vi "YZ_Stage_Movement.vi"(9 "Z Input":dbl, 10 "Y Input":dbl, 11 "X Input":dbl) -> (1 "Current Z Position":sgl, 2 "Current Y Position":sgl, 3 "Current X Position":sgl)   [LabVIEW 2013]
panel:
  out "Original Z Position":sgl
  out "Original Y Position":sgl
  out "Original X Position":sgl
  in  "Z Stage Serial":i32
  in  "Y Stage Serial":i32
  in  "X Stage Serial":i32
  in  "Z Stage Motor":refnum<k7>(container)
  in  "Y Stage Motor":refnum<k7>(container)
  in  "X Stage motor":refnum<k7>(container)
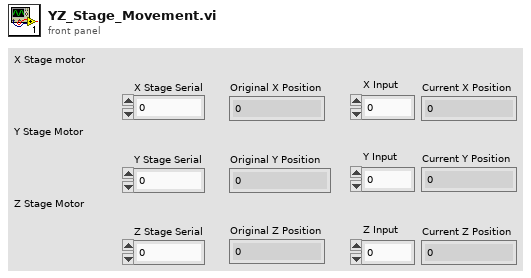
[diagram p1: front panel]
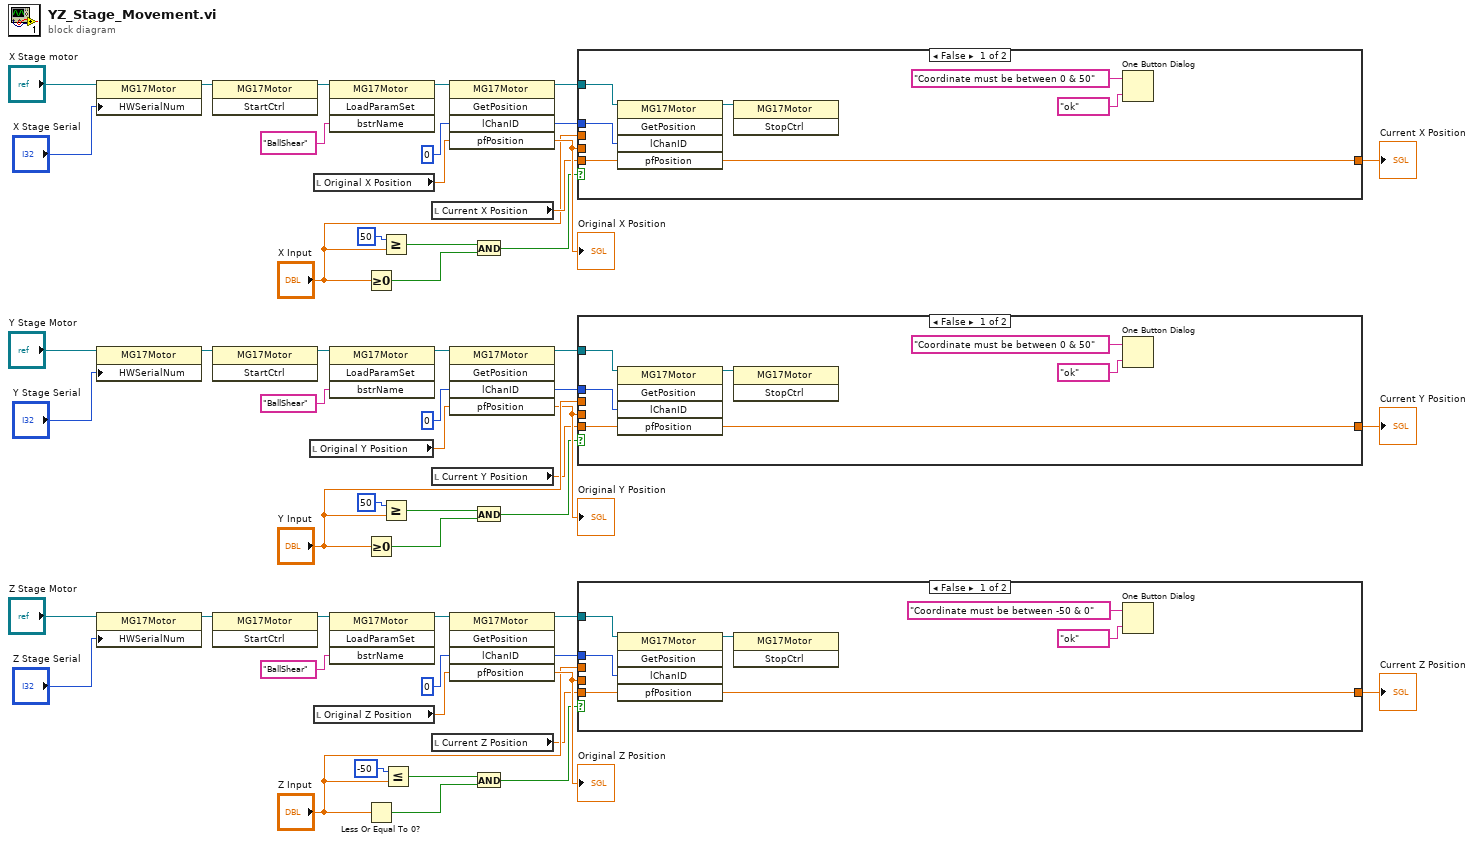
[diagram p0: block diagram]
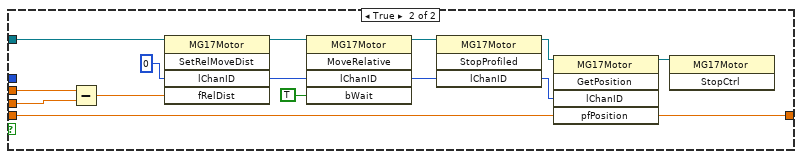
[diagram p2: hidden frame]
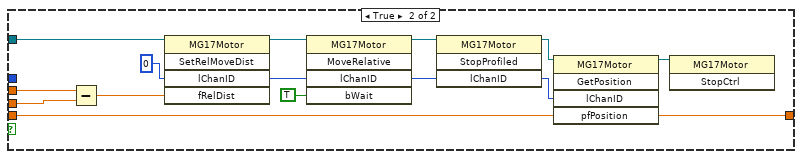
[diagram p3: hidden frame]
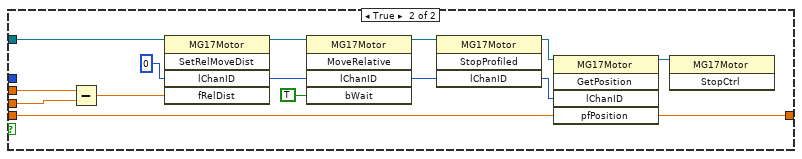
[diagram p4: hidden frame]
diagram:
  n1 = property class="MG17Motor"(reference="X Stage motor", "HWSerialNum"="X Stage Serial") -> (reference out=w46:refnum<k7>)  [unwired: 1 in, 1 out]
  n2 = property class="MG17Motor"(reference="Y Stage Motor", "HWSerialNum"="Y Stage Serial") -> (reference out=w47:refnum<k7>)  [unwired: 1 in, 1 out]
  n3 = property class="MG17Motor"(reference="Z Stage Motor", "HWSerialNum"="Z Stage Serial") -> (reference out=w48:refnum<k7>)  [unwired: 1 in, 1 out]
  n4 = invoke class="MG17Motor" method="StartCtrl"(reference=w46) -> (reference out=w16:refnum<k7>)  [unwired: 2 in, 2 out]
  n5 = invoke class="MG17Motor" method="StartCtrl"(reference=w47) -> (reference out=w13:refnum<k7>)  [unwired: 2 in, 2 out]
  n6 = invoke class="MG17Motor" method="StartCtrl"(reference=w48) -> (reference out=w18:refnum<k7>)  [unwired: 2 in, 2 out]
  n7 = local read "Original Y Position"() -> (w36:sgl)
  n8 = local read "Original X Position"() -> (w44:sgl)
  n9 = local read "Original Z Position"() -> (w28:sgl)
  n10 = invoke class="MG17Motor" method="LoadParamSet"(reference=w16, "bstrName"="BallShear") -> (reference out=w15:refnum<k7>)  [unwired: 2 in, 3 out]
  n11 = invoke class="MG17Motor" method="LoadParamSet"(reference=w13, "bstrName"="BallShear") -> (reference out=w12:refnum<k7>)  [unwired: 2 in, 3 out]
  n12 = invoke class="MG17Motor" method="LoadParamSet"(reference=w18, "bstrName"="BallShear") -> (reference out=w19:refnum<k7>)  [unwired: 2 in, 3 out]
  n13 = Greater Or Equal To 0?(x="X Input") -> (x >= 0?=w43:bool)
  n14 = Greater Or Equal To 0?(x="Y Input") -> (x >= 0?=w35:bool)
  n15 = Less Or Equal To 0?(x="Z Input") -> (x <= 0?=w21:bool)
  n16 = Greater Or Equal?(x=50, y="X Input") -> (x >= y?=w42:bool)
  n17 = Greater Or Equal?(x=50, y="Y Input") -> (x >= y?=w34:bool)
  n18 = Less Or Equal?(x=-50, y="Z Input") -> (x <= y?=w23:bool)
  n19 = local read "Current X Position"() -> (w10:sgl)
  n20 = local read "Current Y Position"() -> (w8:sgl)
  n21 = local read "Current Z Position"() -> (w6:sgl)
  n22 = invoke class="MG17Motor" method="GetPosition"(reference=w15, "lChanID"=0, "pfPosition"=w44) -> (reference out=w38:refnum<k7>, "lChanID"=w2:i32, "pfPosition"=w40:sgl)  [unwired: 2 in, 2 out]
  "Original X Position" <- w40
  n23 = invoke class="MG17Motor" method="GetPosition"(reference=w12, "lChanID"=0, "pfPosition"=w36) -> (reference out=w30:refnum<k7>, "lChanID"=w4:i32, "pfPosition"=w31:sgl)  [unwired: 2 in, 2 out]
  "Original Y Position" <- w31
  n24 = invoke class="MG17Motor" method="GetPosition"(reference=w19, "lChanID"=0, "pfPosition"=w28) -> (reference out=w25:refnum<k7>, "lChanID"=w3:i32, "pfPosition"=w27:sgl)  [unwired: 2 in, 2 out]
  "Original Z Position" <- w27
  n25 = And(x=w42, y=w43) -> (x .and. y?=w39:bool)
  n26 = And(x=w34, y=w35) -> (x .and. y?=w11:bool)
  n27 = And(x=w23, y=w21) -> (x .and. y?=w26:bool)
  n28 = case shown="False" w39 {
    tunnel: "X Input" -> [_ w68]
    tunnel: w40 -> [_ w67]
    tunnel: w38 -> [w59 w69]
    tunnel: w10 -> [w57 w64]
    tunnel: [w56 w63] -> w9
    tunnel: w2 -> [w55 _]
    frame False {
      n29 = invoke class="MG17Motor" method="GetPosition"(reference=w59, "lChanID"=w55, "pfPosition"=w57) -> (reference out=w58:refnum<k7>, "pfPosition"=w56:sgl)  [unwired: 2 in, 3 out]
      n30 = invoke class="MG17Motor" method="StopCtrl"(reference=w58) -> ()  [unwired: 2 in, 3 out]
      n31 = One Button Dialog(message="Coordinate must be between 0 & 50", button name ("OK")="ok") -> ()  [unwired: 1 out]
    }
    frame True {
      n32 = Subtract(x=w68, y=w67) -> (x-y=w70:dbl)
      n33 = invoke class="MG17Motor" method="SetRelMoveDist"(reference=w69, "lChanID"=0, "fRelDist"=w70) -> (reference out=w73:refnum<k7>, "lChanID"=w74:i32)  [unwired: 2 in, 3 out]
      n34 = invoke class="MG17Motor" method="MoveRelative"(reference=w73, "lChanID"=w74, "bWait"=TRUE) -> (reference out=w75:refnum<k7>, "lChanID"=w76:i32)  [unwired: 2 in, 3 out]
      n35 = invoke class="MG17Motor" method="StopProfiled"(reference=w75, "lChanID"=w76) -> (reference out=w66:refnum<k7>, "lChanID"=w62:i32)  [unwired: 2 in, 2 out]
      n36 = invoke class="MG17Motor" method="GetPosition"(reference=w66, "lChanID"=w62, "pfPosition"=w64) -> (reference out=w65:refnum<k7>, "pfPosition"=w63:sgl)  [unwired: 2 in, 3 out]
      n37 = invoke class="MG17Motor" method="StopCtrl"(reference=w65) -> ()  [unwired: 2 in, 3 out]
    }
  }
  "Current X Position" <- w9
  n38 = case shown="False" w11 {
    tunnel: "Y Input" -> [_ w89]
    tunnel: w31 -> [_ w90]
    tunnel: w30 -> [w83 w91]
    tunnel: w8 -> [w79 w85]
    tunnel: [w78 w84] -> w7
    tunnel: w4 -> [w77 _]
    frame False {
      n39 = invoke class="MG17Motor" method="GetPosition"(reference=w83, "lChanID"=w77, "pfPosition"=w79) -> (reference out=w80:refnum<k7>, "pfPosition"=w78:sgl)  [unwired: 2 in, 3 out]
      n40 = invoke class="MG17Motor" method="StopCtrl"(reference=w80) -> ()  [unwired: 2 in, 3 out]
      n41 = One Button Dialog(message="Coordinate must be between 0 & 50", button name ("OK")="ok") -> ()  [unwired: 1 out]
    }
    frame True {
      n42 = Subtract(x=w89, y=w90) -> (x-y=w92:dbl)
      n43 = invoke class="MG17Motor" method="SetRelMoveDist"(reference=w91, "lChanID"=0, "fRelDist"=w92) -> (reference out=w95:refnum<k7>, "lChanID"=w96:i32)  [unwired: 2 in, 3 out]
      n44 = invoke class="MG17Motor" method="MoveRelative"(reference=w95, "lChanID"=w96, "bWait"=TRUE) -> (reference out=w97:refnum<k7>, "lChanID"=w98:i32)  [unwired: 2 in, 3 out]
      n45 = invoke class="MG17Motor" method="StopProfiled"(reference=w97, "lChanID"=w98) -> (reference out=w88:refnum<k7>, "lChanID"=w86:i32)  [unwired: 2 in, 2 out]
      n46 = invoke class="MG17Motor" method="GetPosition"(reference=w88, "lChanID"=w86, "pfPosition"=w85) -> (reference out=w87:refnum<k7>, "pfPosition"=w84:sgl)  [unwired: 2 in, 3 out]
      n47 = invoke class="MG17Motor" method="StopCtrl"(reference=w87) -> ()  [unwired: 2 in, 3 out]
    }
  }
  "Current Y Position" <- w7
  n48 = case shown="False" w26 {
    tunnel: "Z Input" -> [_ w111]
    tunnel: w27 -> [_ w112]
    tunnel: w25 -> [w105 w113]
    tunnel: [w101 w108] -> w5
    tunnel: w6 -> [w102 w107]
    tunnel: w3 -> [w99 _]
    frame False {
      n49 = invoke class="MG17Motor" method="GetPosition"(reference=w105, "lChanID"=w99, "pfPosition"=w102) -> (reference out=w100:refnum<k7>, "pfPosition"=w101:sgl)  [unwired: 2 in, 3 out]
      n50 = invoke class="MG17Motor" method="StopCtrl"(reference=w100) -> ()  [unwired: 2 in, 3 out]
      n51 = One Button Dialog(message="Coordinate must be between -50 & 0", button name ("OK")="ok") -> ()  [unwired: 1 out]
    }
    frame True {
      n52 = Subtract(x=w111, y=w112) -> (x-y=w114:dbl)
      n53 = invoke class="MG17Motor" method="SetRelMoveDist"(reference=w113, "lChanID"=0, "fRelDist"=w114) -> (reference out=w117:refnum<k7>, "lChanID"=w118:i32)  [unwired: 2 in, 3 out]
      n54 = invoke class="MG17Motor" method="MoveRelative"(reference=w117, "lChanID"=w118, "bWait"=TRUE) -> (reference out=w119:refnum<k7>, "lChanID"=w120:i32)  [unwired: 2 in, 3 out]
      n55 = invoke class="MG17Motor" method="StopProfiled"(reference=w119, "lChanID"=w120) -> (reference out=w106:refnum<k7>, "lChanID"=w110:i32)  [unwired: 2 in, 2 out]
      n56 = invoke class="MG17Motor" method="GetPosition"(reference=w106, "lChanID"=w110, "pfPosition"=w107) -> (reference out=w109:refnum<k7>, "pfPosition"=w108:sgl)  [unwired: 2 in, 3 out]
      n57 = invoke class="MG17Motor" method="StopCtrl"(reference=w109) -> ()  [unwired: 2 in, 3 out]
    }
  }
  "Current Z Position" <- w5
